vi "数据表比对.vi"(8 "error in (no error)":errorcluster, 9 "查询元素输入":string(combo), 10 "仪器日志参数":string, 11 "table输入":string(combo)) -> (0 "error out":errorcluster, 2 "待发送第一条数据":string[](array[string]), 3 "待发送数据":string[][](table))   [LabVIEW 2016, in "数据传输系统.lvlib"]
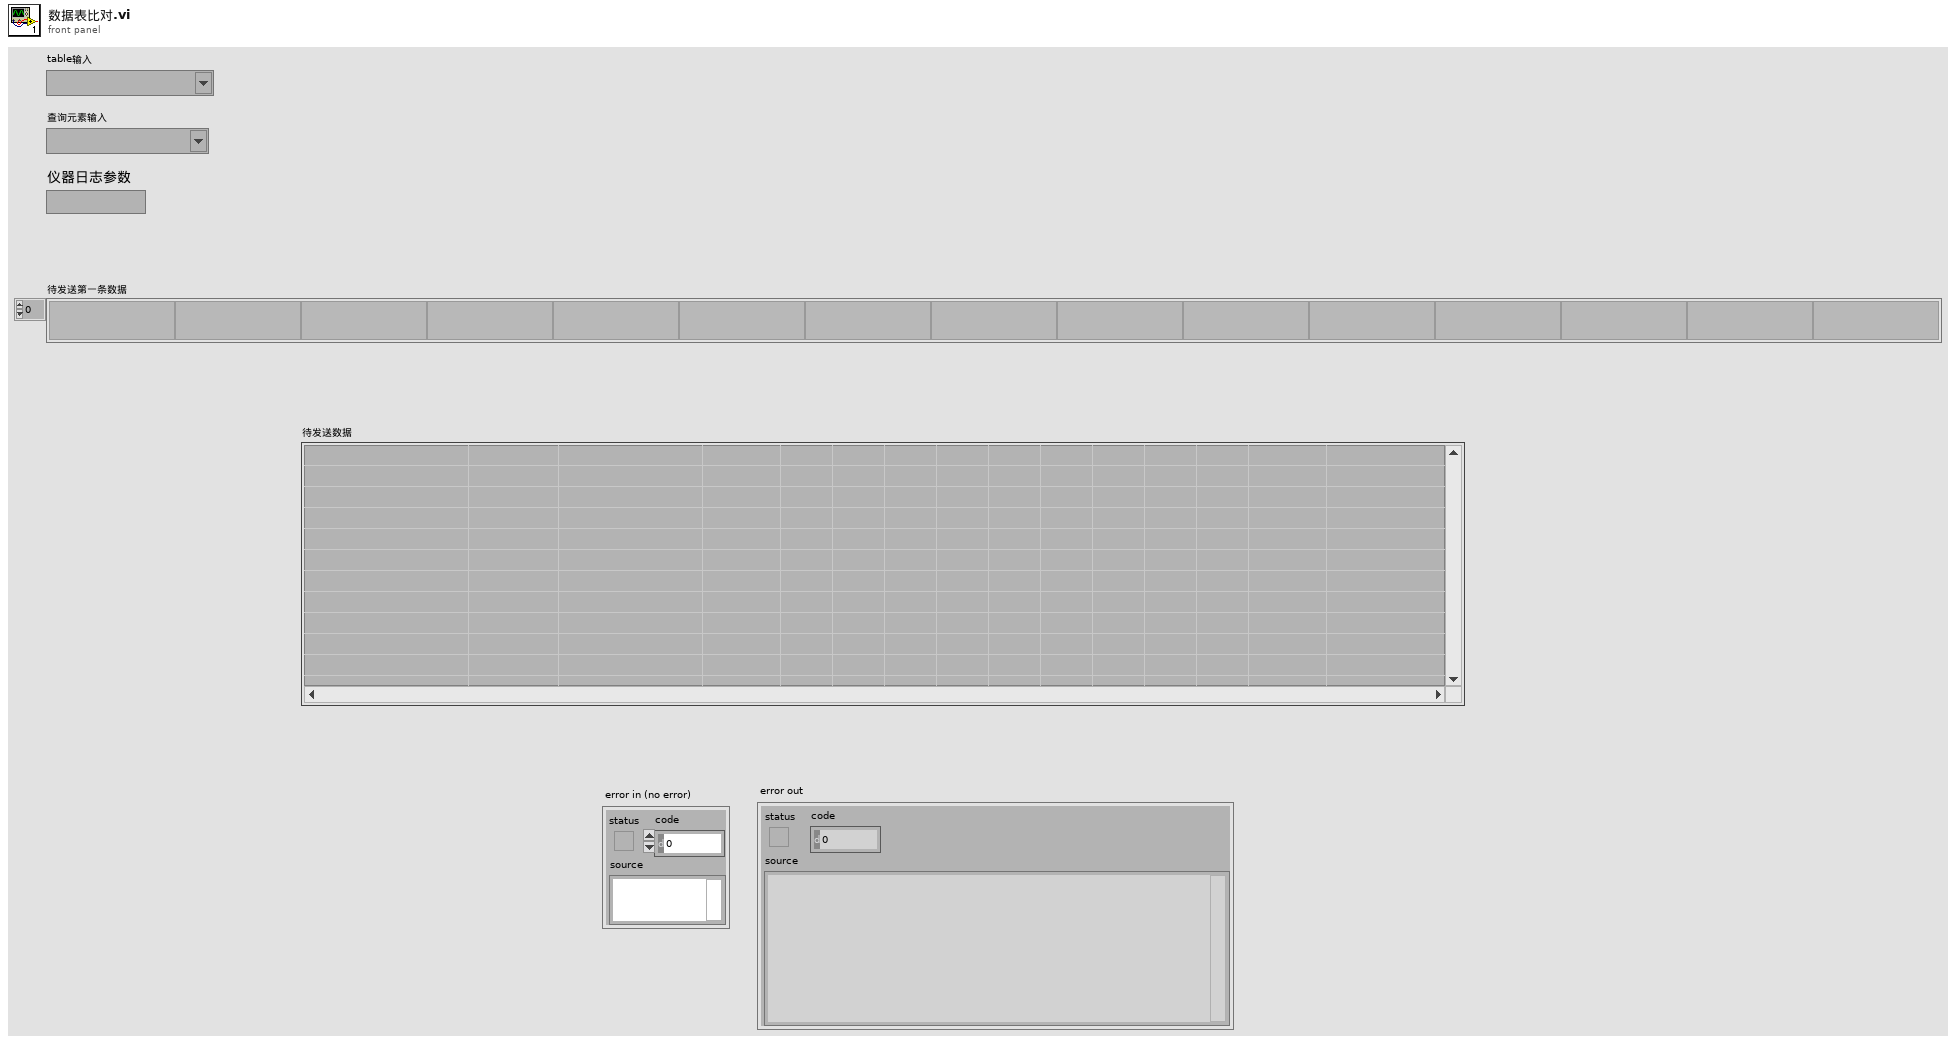
[diagram p1: front panel]
types:
  T1 = typedef "LVDateTimeRec.ctl" = cluster{"秒数的小数部分":dbl, "秒":i32, "分":i32, "时":i32, "日":i32, "月":i32, "年":i32, "天数（周）":i32, "天数（年）":i32, "DST":i32}
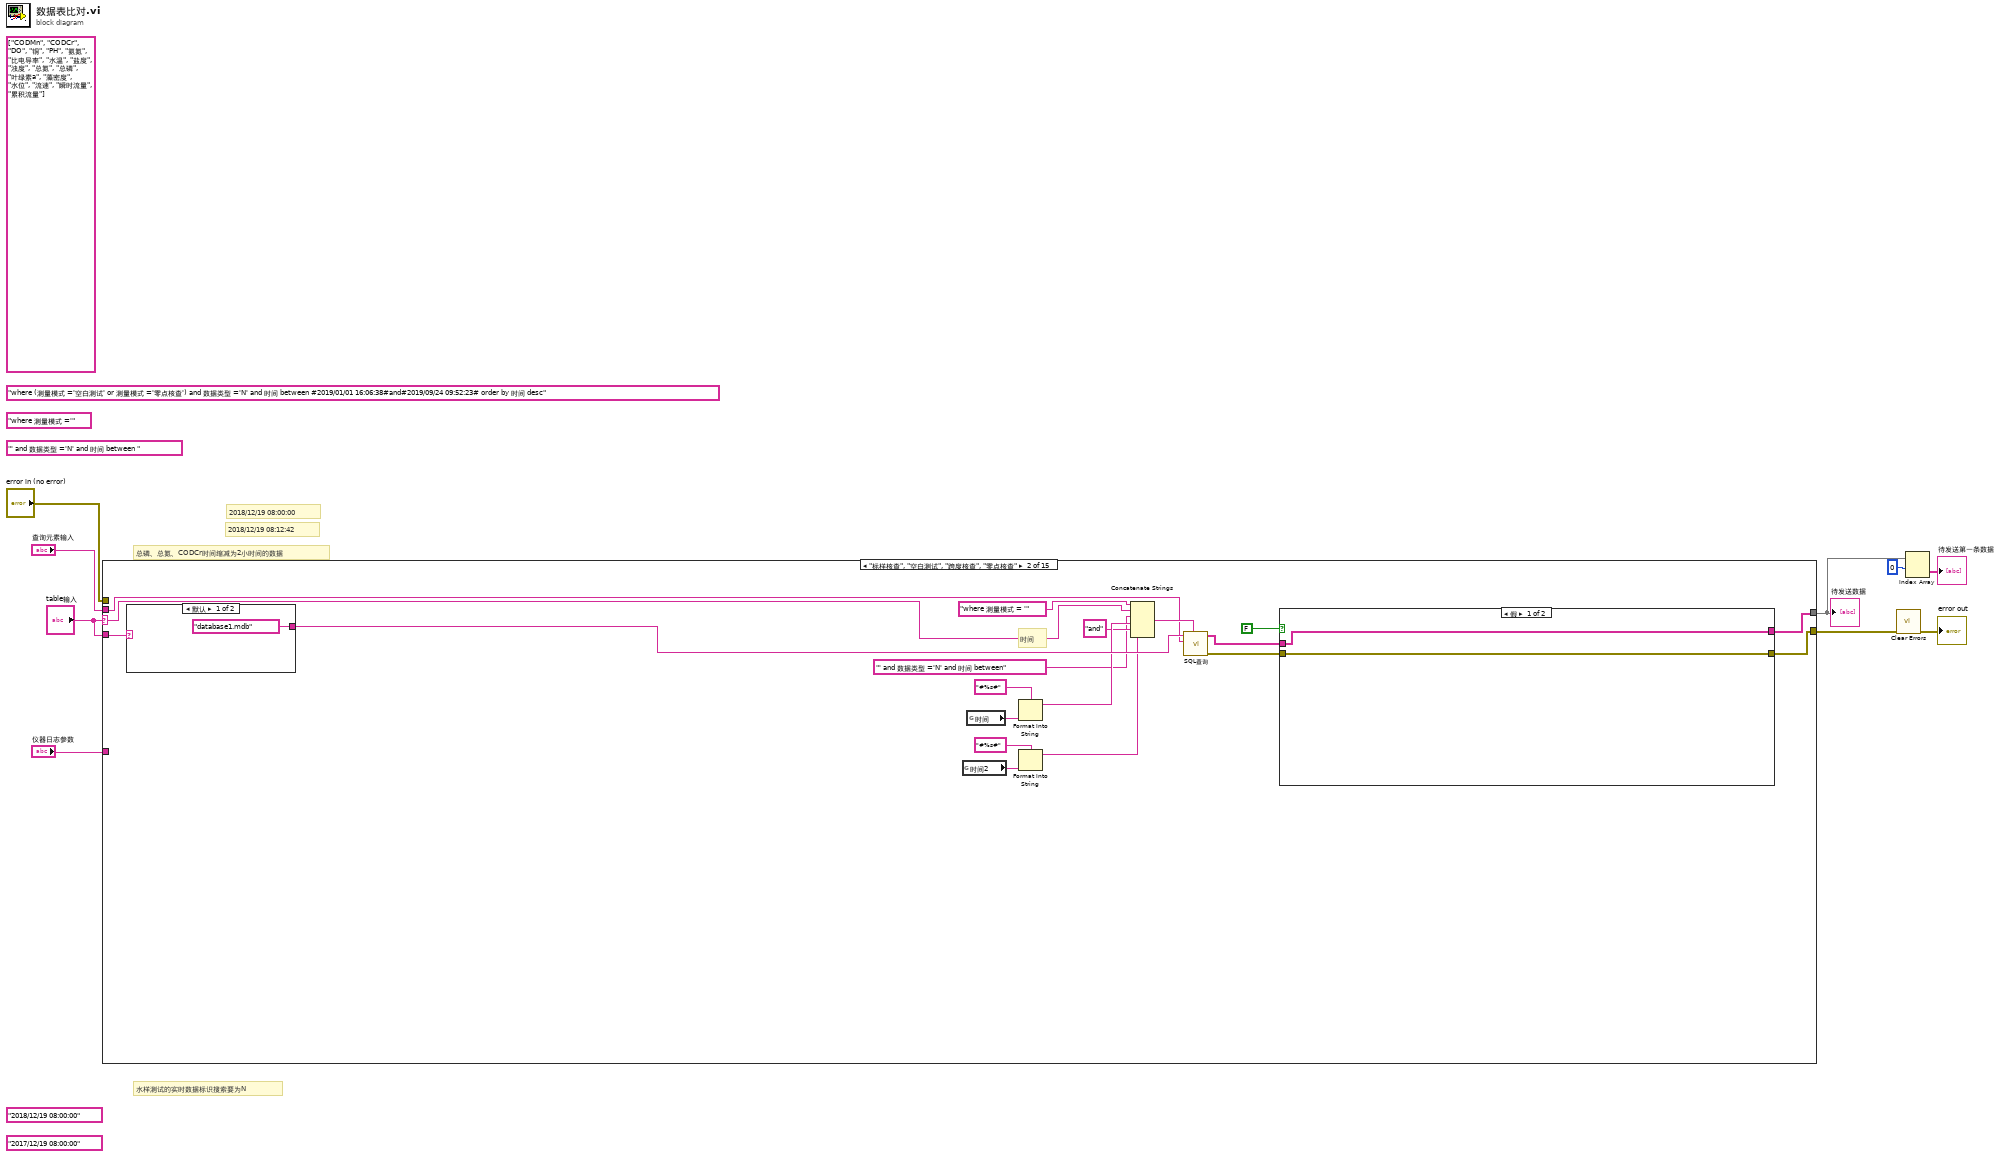
[diagram p0: block diagram]
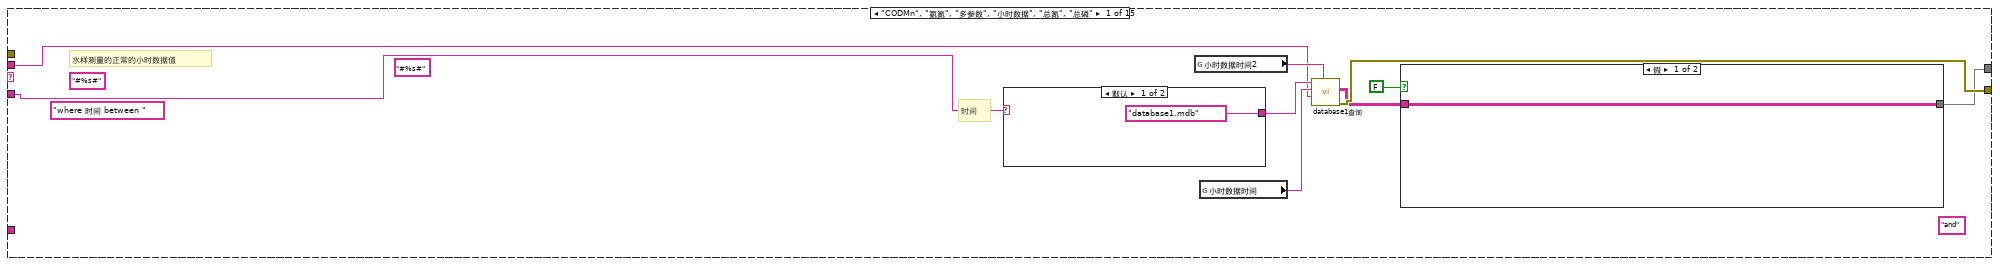
[diagram p2: hidden frame]
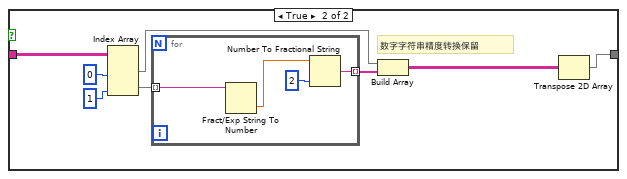
[diagram p3: hidden frame]
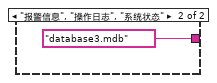
[diagram p4: hidden frame]
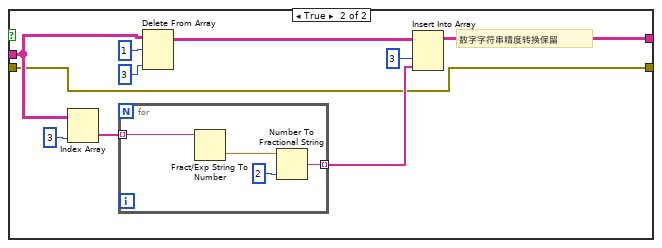
[diagram p5: hidden frame]
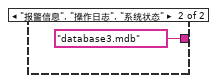
[diagram p6: hidden frame]
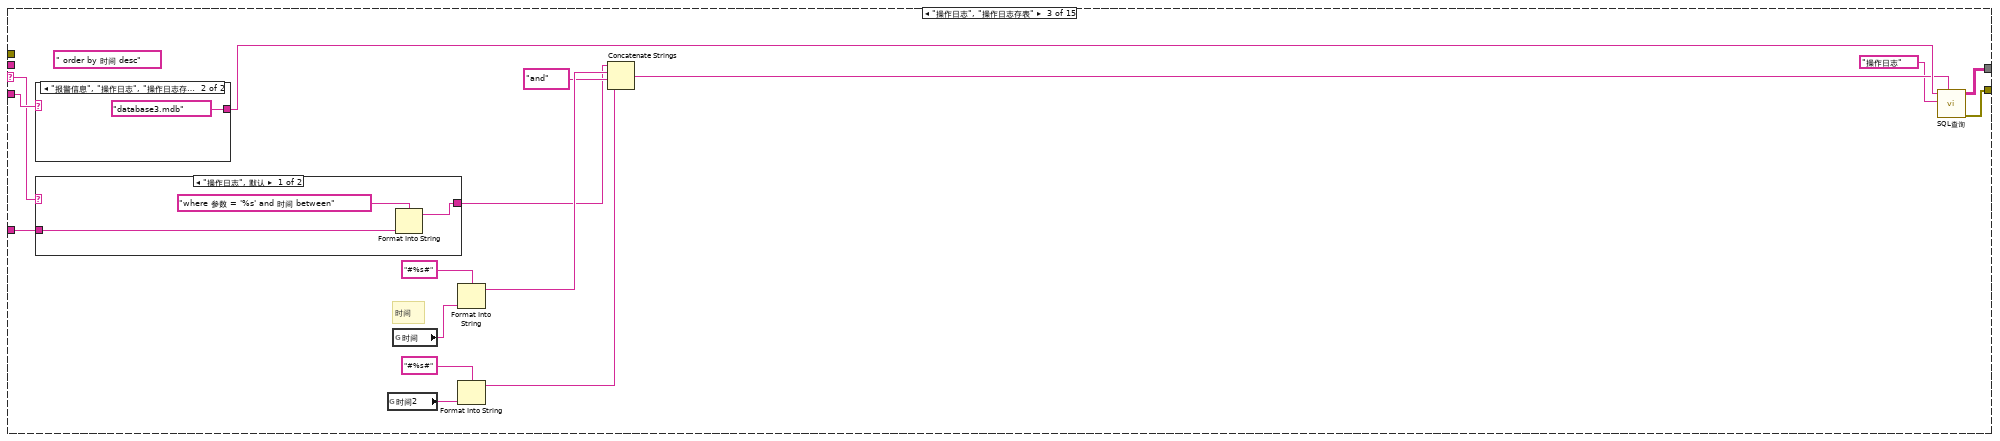
[diagram p7: hidden frame]
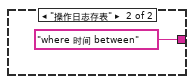
[diagram p8: hidden frame]
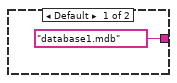
[diagram p9: hidden frame]
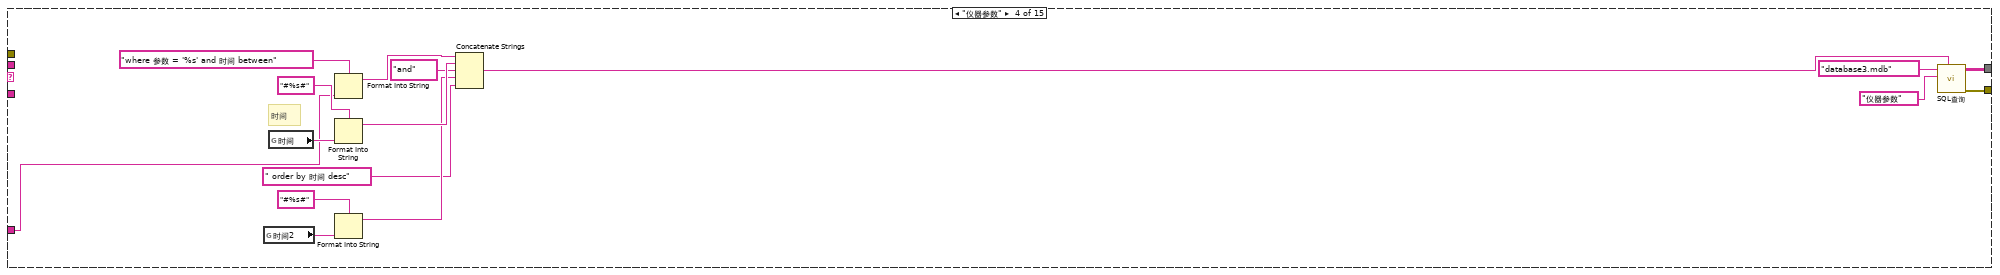
[diagram p10: hidden frame]
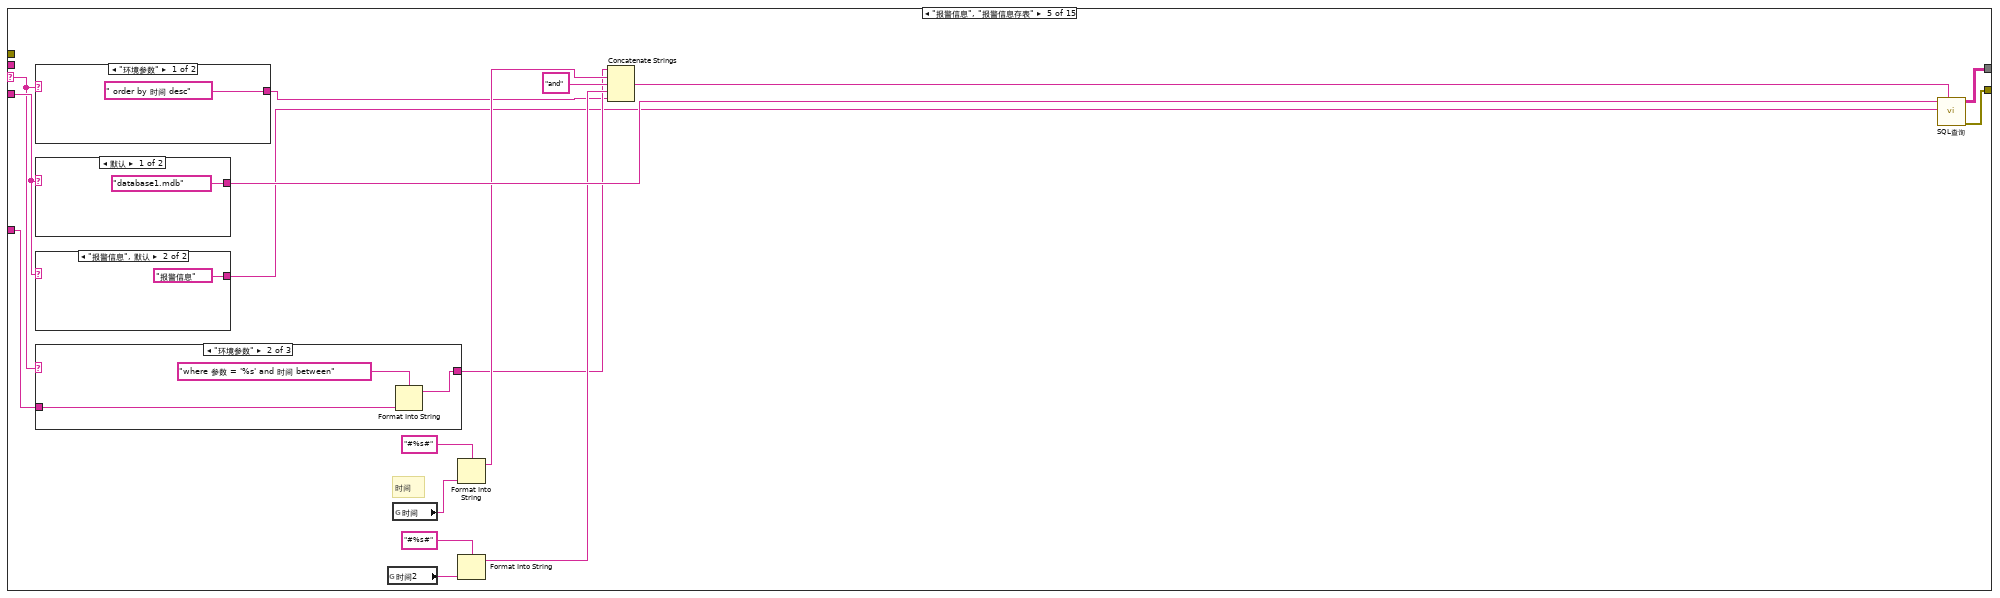
[diagram p11: hidden frame]
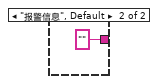
[diagram p12: hidden frame]
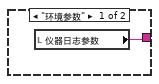
[diagram p13: hidden frame]
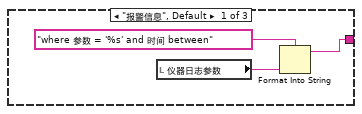
[diagram p14: hidden frame]
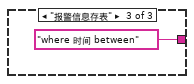
[diagram p15: hidden frame]
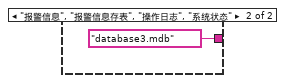
[diagram p16: hidden frame]
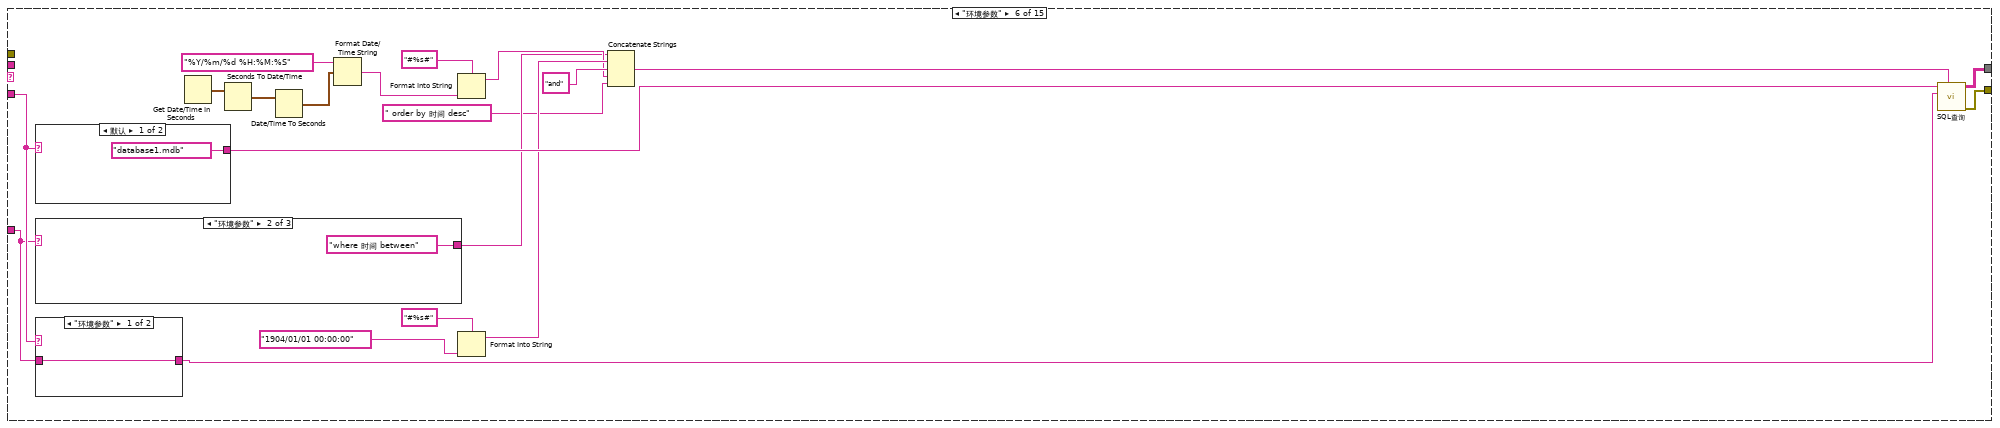
[diagram p17: hidden frame]
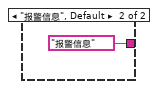
[diagram p18: hidden frame]
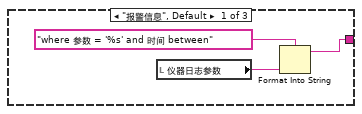
[diagram p19: hidden frame]
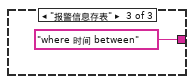
[diagram p20: hidden frame]
diagram:
  (unwired) "' and 数据类型 ='N' and 时间 between "
  (unwired) "where 测量模式 ='" ("condition")
  (unwired) "where (测量模式 ='空白测试' or 测量模式 ='零点核查') and 数据类型 ='N' and 时间 between #2019/01/01 16:06:38#and#2019/09/24 09:52:23# order by 时间 desc" ("condition")
  (unwired) string[] ["CODMn", "CODCr", "DO", "铜", "PH", "氨氮", "比电导率", "水温", "盐度", "浊度", "总氮", "总磷", "叶绿素a", "藻密度", "水位", "流速", "瞬时流量", "累积流量"] ("查询参数数组")
  (unwired) "2017/12/19 08:00:00"
  (unwired) "2018/12/19 08:00:00"
  # "水样测试的实时数据标识搜索要为N"
  # "2018/12/19 08:00:00"
  # "总磷、总氮、CODCr时间缩减为2小时间的数据"
  # "2018/12/19 08:12:42"
  n1 = case shown="\"标样核查\", \"空白测试\", \"跨度核查\", \"零点核查\"" "table输入" {
    selector: "table输入" -> [_ w35 w72 _ w109 _ _ _ _ _ _ _ _ _ _]
    tunnel: "error in (no error)" -> [_ _ _ _ _ _ w170 _ _ _ _ _ _ _ _]
    tunnel: [w16 w38 w84 w107 w124 w157 w170 w185 w281 w328 w382 w437 w480 w523 w564] -> w7
    tunnel: [w12 w41 w82 w105 w122 w155 w168 w188 w284 w331 w385 w440 w483 w526 w566] -> w3
    tunnel: "table输入" -> [w18 w52 w86 _ w112 w147 _ _ _ _ _ _ _ _ _]
    tunnel: "查询元素输入" -> [w10 w34 _ _ _ _ _ w171 w270 w317 w371 w430 w473 w516 w559]
    tunnel: "仪器日志参数" -> [_ _ w71 w93 w110 w139 _ _ _ _ _ _ _ _ _]
    frame "CODMn", "氨氮", "多参数", "小时数据", "总氮", "总磷" {
      (unwired) "and" ("字符串")
      (unwired) "#%s#" ("初始字符串")
      (unwired) "#%s#" ("初始字符串")
      (unwired) "where 时间 between " ("condition")
      # "水样测量的正常的小时数据值"
      # "时间"
      n2 = case shown="默认" w18 {
        tunnel: ["database1.mdb" ("database") "database3.mdb" ("database")] -> w17
        frame Default {
        }
        frame "报警信息", "操作日志", "系统状态" {
        }
      }
      n3 = global read "全局 时间2.vi" "小时数据时间2"() -> (w14:string)
      n4 = global read "全局 水样时间.vi" "小时数据时间"() -> (w15:string)
      n5 = call "database1查询.vi"("时间2"=w14, "table"=w10, "时间1"=w15, "database"=w17) -> ("error out"=w16:errorcluster, "data"=w13:string[][])  [unwired: 4 in, 1 out]
      n6 = case shown="假" FALSE {
        tunnel: w13 -> [w19 w27]
        tunnel: [w19 w20] -> w12
        frame False {
        }
        frame True {
          # "数字字符串精度转换保留"
          n7 = Index Array(array=w27, index (col) #1=0 ("禁用的索引 (列)"), index (col) #2=1 ("索引 (列)")) -> (element #1=w23:string[], element #2=w24:string[])  [unwired: 2 in]
          n8 = for {
            tunnel: w24 -> [w29] mode=indexing
            tunnel: [w28] -> w22 mode=indexing
            n9 = Fract/Exp String To Number(string=w29) -> (number=w30:dbl)  [unwired: 3 in, 1 out]
            n10 = Number To Fractional String(number=w30, precision (6)=i16 2 ("精度(6)")) -> (F-format string=w28:string)  [unwired: 2 in]
          }
          n11 = Build Array(w23, w22) -> (w21:string[][])
          n12 = Transpose 2D Array(2D array=w21) -> (transposed array=w20:string[][])
        }
      }
    }
    frame "标样核查", "空白测试", "跨度核查", "零点核查" {
      # "时间"
      n13 = case shown="默认" w52 {
        tunnel: ["database1.mdb" ("database") "database3.mdb" ("database")] -> w51
        frame Default {
        }
        frame "报警信息", "操作日志", "系统状态" {
        }
      }
      n14 = global read "全局 时间2.vi" "时间2"() -> (w43:string)
      n15 = global read "全局 水样时间.vi" "时间"() -> (w44:string)
      n16 = Format Into String(format string="#%s#" ("初始字符串"), w44) -> (resulting string=w50:string)  [unwired: 2 in, 1 out]
      n17 = Format Into String(format string="#%s#" ("初始字符串"), w43) -> (resulting string=w46:string)  [unwired: 2 in, 1 out]
      n18 = Concatenate Strings("where 测量模式 = '" ("condition"), w35, "' and 数据类型 ='N' and 时间 between" ("字符串"), w50, "and" ("字符串"), w46) -> (w45:string)
      n19 = call "SQL查询.vi"("condition"=w45, "table输入"=w34, "database"=w51) -> ("error out"=w39:errorcluster, "data"=w42:string[][])  [unwired: 7 in]
      n20 = case shown="假" FALSE {
        tunnel: w42 -> [w54 w57]
        tunnel: [w54 w56] -> w41
        tunnel: [w53 w55] -> w38
        tunnel: w39 -> [w53 w55]
        frame False {
        }
        frame True {
          # "数字字符串精度转换保留"
          n21 = Index Array(array=w57, index (col)=3 ("禁用的索引 (列)")) -> (element=w63:string[])  [unwired: 1 in]
          n22 = for {
            tunnel: w63 -> [w66] mode=indexing
            tunnel: [w65] -> w59 mode=indexing
            n23 = Fract/Exp String To Number(string=w66) -> (number=w67:dbl)  [unwired: 3 in, 1 out]
            n24 = Number To Fractional String(number=w67, precision (6)=i16 2 ("精度(6)")) -> (F-format string=w65:string)  [unwired: 2 in]
          }
          n25 = Delete From Array(array=w57, length=1 ("长度"), index (col)=3 ("禁用的索引 (列)")) -> (array with subset deleted=w60:string[][])  [unwired: 1 in, 1 out]
          n26 = Insert Into Array(array=w60, index (col)=3 ("禁用的索引 (列)"), new element=w59) -> (w56:string[][])  [unwired: 1 in]
        }
      }
    }
    frame "操作日志", "操作日志存表" {
      (unwired) " order by 时间 desc" ("字符串")
      # "时间"
      n27 = case shown="\"报警信息\", \"操作日志\", \"操作日志存表\", \"系统状态\"" w86 {
        tunnel: ["database1.mdb" ("database") "database3.mdb" ("database")] -> w85
        frame Default {
        }
        frame "报警信息", "操作日志", "操作日志存表", "系统状态" {
        }
      }
      n28 = case shown="\"操作日志\", 默认" w72 {
        tunnel: [w88 "where 时间 between" ("condition")] -> w74
        tunnel: w71 -> [w87 _]
        frame "操作日志", Default {
          n29 = Format Into String(format string="where 参数 = '%s' and 时间 between" ("condition"), w87) -> (resulting string=w88:string)  [unwired: 2 in, 1 out]
        }
        frame "操作日志存表" {
        }
      }
      n30 = global read "全局 时间2.vi" "时间2"() -> (w75:string)
      n31 = global read "全局 水样时间.vi" "时间"() -> (w76:string)
      n32 = Format Into String(format string="#%s#" ("初始字符串"), w76) -> (resulting string=w81:string)  [unwired: 2 in, 1 out]
      n33 = Format Into String(format string="#%s#" ("初始字符串"), w75) -> (resulting string=w77:string)  [unwired: 2 in, 1 out]
      n34 = Concatenate Strings(w74, w81, "and" ("字符串"), w77) -> (w83:string)
      n35 = call "SQL查询.vi"("condition"=w83, "table输入"="操作日志", "database"=w85) -> ("error out"=w84:errorcluster, "data"=w82:string[][])  [unwired: 7 in]
    }
    frame "仪器参数" {
      # "时间"
      n36 = global read "全局 时间2.vi" "时间2"() -> (w98:string)
      n37 = global read "全局 水样时间.vi" "时间"() -> (w99:string)
      n38 = Format Into String(format string="where 参数 = '%s' and 时间 between" ("condition"), w93) -> (resulting string=w97:string)  [unwired: 2 in, 1 out]
      n39 = Format Into String(format string="#%s#" ("初始字符串"), w99) -> (resulting string=w104:string)  [unwired: 2 in, 1 out]
      n40 = Format Into String(format string="#%s#" ("初始字符串"), w98) -> (resulting string=w100:string)  [unwired: 2 in, 1 out]
      n41 = Concatenate Strings(w97, w104, "and" ("字符串"), w100, " order by 时间 desc" ("字符串")) -> (w106:string)
      n42 = call "SQL查询.vi"("condition"=w106, "table输入"="仪器参数", "database"="database3.mdb") -> ("error out"=w107:errorcluster, "data"=w105:string[][])  [unwired: 7 in]
    }
    frame "报警信息", "报警信息存表" {
      # "时间"
      n43 = case shown="\"环境参数\"" w109 {
        tunnel: [" order by 时间 desc" ("字符串") "" ("仪器日志参数")] -> w111
        frame "环境参数" {
        }
        frame "报警信息", Default {
        }
      }
      n44 = case shown="默认" w112 {
        tunnel: ["database1.mdb" ("database") "database3.mdb" ("database")] -> w125
        frame Default {
        }
        frame "报警信息", "报警信息存表", "操作日志", "系统状态" {
        }
      }
      n45 = case shown="\"报警信息\", 默认" w112 {
        tunnel: [w128 "报警信息" ("table输入")] -> w113
        frame "环境参数" {
          n46 = local read "仪器日志参数"() -> (w128:string)
        }
        frame "报警信息", Default {
        }
      }
      n47 = case shown="\"环境参数\"" w109 {
        tunnel: [w131 w134 "where 时间 between" ("condition")] -> w114
        tunnel: w110 -> [_ w133 _]
        frame "报警信息", Default {
          n48 = local read "仪器日志参数"() -> (w130:string)
          n49 = Format Into String(format string="where 参数 = '%s' and 时间 between" ("condition"), w130) -> (resulting string=w131:string)  [unwired: 2 in, 1 out]
        }
        frame "环境参数" {
          n50 = Format Into String(format string="where 参数 = '%s' and 时间 between" ("condition"), w133) -> (resulting string=w134:string)  [unwired: 2 in, 1 out]
        }
        frame "报警信息存表" {
        }
      }
      n51 = global read "全局 时间2.vi" "时间2"() -> (w115:string)
      n52 = global read "全局 水样时间.vi" "时间"() -> (w116:string)
      n53 = Format Into String(format string="#%s#" ("初始字符串"), w116) -> (resulting string=w121:string)  [unwired: 2 in, 1 out]
      n54 = Format Into String(format string="#%s#" ("初始字符串"), w115) -> (resulting string=w117:string)  [unwired: 2 in, 1 out]
      n55 = Concatenate Strings(w114, w121, "and" ("字符串"), w117, w111) -> (w123:string)
      n56 = call "SQL查询.vi"("condition"=w123, "table输入"=w113, "database"=w125) -> ("error out"=w124:errorcluster, "data"=w122:string[][])  [unwired: 7 in]
    }
    frame "环境参数" {
      n57 = case shown="默认" w147 {
        tunnel: ["database1.mdb" ("database") "database3.mdb" ("database")] -> w158
        frame Default {
        }
        frame "报警信息", "报警信息存表", "操作日志", "系统状态" {
        }
      }
      n58 = case shown="\"环境参数\"" w139 {
        tunnel: [w162 "where 时间 between" ("condition") "where 时间 between" ("condition")] -> w149
        frame "报警信息", Default {
          n59 = local read "仪器日志参数"() -> (w161:string)
          n60 = Format Into String(format string="where 参数 = '%s' and 时间 between" ("condition"), w161) -> (resulting string=w162:string)  [unwired: 2 in, 1 out]
        }
        frame "环境参数" {
        }
        frame "报警信息存表" {
        }
      }
      n61 = case shown="\"环境参数\"" w147 {
        tunnel: [w159 "报警信息" ("table输入")] -> w148
        tunnel: w139 -> [w159 _]
        frame "环境参数" {
        }
        frame "报警信息", Default {
        }
      }
      n62 = Get Date/Time In Seconds() -> (seconds since 1Jan1904=w144:timestamp)
      n63 = Seconds To Date/Time(time stamp (now)=w144) -> (date time rec=w141:T1)  [unwired: 1 in]
      n64 = Date/Time To Seconds(2:w141) -> (0:w143:timestamp)  [unwired: 1 in]
      n65 = Format Date/Time String(time format string (%c)="%Y/%m/%d %H:%M:%S" ("时间格式字符串(%c)"), seconds (now)=w143) -> (date/time string=w140:string)  [unwired: 1 in]
      n66 = Format Into String(format string="#%s#" ("初始字符串"), w140) -> (resulting string=w150:string)  [unwired: 2 in, 1 out]
      n67 = Format Into String(format string="#%s#" ("初始字符串"), "1904/01/01 00:00:00") -> (resulting string=w154:string)  [unwired: 2 in, 1 out]
      n68 = Concatenate Strings(w149, w154, "and" ("字符串"), w150, " order by 时间 desc" ("字符串")) -> (w156:string)
      n69 = call "SQL查询.vi"("condition"=w156, "table输入"=w148, "database"=w158) -> ("error out"=w157:errorcluster, "data"=w155:string[][])  [unwired: 7 in]
    }
    frame Default {
      # "时间格式转换"
      n70 = local read "待发送数据"() -> (w169:string[][])
      n71 = call "数组时间戳格式化(子VI).vi"("待发送数据输入"=w169) -> ("待发送数据输出"=w168:string[][])  [unwired: 10 in]
    }
    frame "实时数据" {
      (unwired) " order by 时间 desc" ("字符串")
      # "空白测试or零点核查要加括号"
      # "上传本地时间点的实时数据"
      # "上传质控数据（空白测试，跨度核查，核查数据，平行样数据）"
      n72 = global read "全局 实时数据参数.vi" "实时数据参数"() -> (w181:string)
      n73 = case shown="\"空白测试\"" w181 {
        tunnel: [w205 w227 w238 w244] -> w182
        tunnel: w181 -> [w201 w226 _ w240]
        tunnel: [w204 w222 w234 w239] -> w176
        tunnel: w171 -> [_ w221 _ _]
        frame "水样测试" {
          n74 = Get Date/Time In Seconds() -> (seconds since 1Jan1904=w213:timestamp)
          n75 = Format Date/Time String(time format string (%c)="%Y%m%d%H%M%S%3u" ("时间格式字符串(%c)"), seconds (now)=w213) -> (date/time string=w211:string)  [unwired: 1 in]
          n76 = local read "查询元素输入"() -> (w206:string)
          n77 = Concatenate Strings("where 测量模式 ='" ("condition"), w201, "' and 数据类型 ='N' and 时间 between ") -> (w204:string)
          n78 = Replace Substring(2:8 ("长度（子字符串长度）"), 3:10 ("偏移量(0)"), 4:"0000" ("子字符串(\"\")"), 5:w211) -> (1:w207:string)  [unwired: 1 out]
          n79 = case shown="默认" w206 {
            tunnel: w207 -> [w215 w218 _]
            tunnel: [w214 w219 w220] -> w205
            frame Default {
              n80 = Search and Replace String(input string=w215, search string="." ("搜索字符串")) -> (result string=w216:string)  [unwired: 6 in, 3 out]
              n81 = call "格式时间字符串.vi"("字符串"=w216) -> ("连接的字符串"=w214:string)  [unwired: 10 in]
            }
            frame "CODCr", "CODMn", "累积流量", "总氮", "总磷" {
              n82 = call "实时数据查询用2小时间的数据.vi"("字符串"=w218) -> ("连接的字符串"=w219:string)  [unwired: 10 in]
            }
            frame "CODCr加标回收率", "CODMn加标回收率", "氨氮加标回收率", "总氮加标回收率", "总磷加标回收率" {
              n83 = global read "全局 时间2.vi" "加标回收索引起始时间"() -> (w220:string)
            }
          }
        }
        frame "空白测试" {
          n84 = case shown="\"氨氮\"" w221 {
            tunnel: [w228 w229 w230 w231 w232 w233] -> w227
            frame "CODMn" {
              n85 = global read "全局 时间2.vi" "CODMn零点核查索引起始时间"() -> (w228:string)
            }
            frame "CODCr" {
              n86 = global read "全局 时间2.vi" "CODCr零点核查索引起始时间"() -> (w229:string)
            }
            frame "氨氮" {
              n87 = global read "全局 时间2.vi" "氨氮零点核查索引起始时间"() -> (w230:string)
            }
            frame "总磷" {
              n88 = global read "全局 时间2.vi" "总磷零点核查索引起始时间"() -> (w231:string)
            }
            frame "总氮" {
              n89 = global read "全局 时间2.vi" "总氮零点核查索引起始时间"() -> (w232:string)
            }
            frame "", Default {
              n90 = global read "全局 时间2.vi" "零点核查索引起始时间"() -> (w233:string)
            }
          }
          n91 = Concatenate Strings("where (测量模式 ='" ("condition"), w226, "' or 测量模式 = '零点核查", "') and 数据类型 ='N' and 时间 between ") -> (w222:string)
        }
        frame "核查数据" {
          n92 = global read "全局 时间2.vi" "标样核查索引起始时间"() -> (w238:string)
          n93 = Concatenate Strings("where 测量模式 ='" ("condition"), "标样核查" ("实时数据参数"), "' and 数据类型 ='N' and 时间 between ") -> (w234:string)
        }
        frame "跨度核查", Default {
          n94 = local read "查询元素输入"() -> (w243:string)
          n95 = Concatenate Strings("where 测量模式 ='" ("condition"), w240, "' and 数据类型 ='N' and 时间 between ") -> (w239:string)
          n96 = case shown="\"氨氮\"" w243 {
            tunnel: [w245 w246 w247 w248 w249 w250] -> w244
            frame "CODMn" {
              n97 = global read "全局 时间2.vi" "CODMn跨度核查索引起始时间"() -> (w245:string)
            }
            frame "CODCr" {
              n98 = global read "全局 时间2.vi" "CODCr跨度核查索引起始时间"() -> (w246:string)
            }
            frame "氨氮" {
              n99 = global read "全局 时间2.vi" "氨氮跨度核查索引起始时间"() -> (w247:string)
            }
            frame "总磷" {
              n100 = global read "全局 时间2.vi" "总磷跨度核查索引起始时间"() -> (w248:string)
            }
            frame "总氮" {
              n101 = global read "全局 时间2.vi" "总氮跨度核查索引起始时间"() -> (w249:string)
            }
            frame "", Default {
              n102 = global read "全局 时间2.vi" "跨度核查索引起始时间"() -> (w250:string)
            }
          }
        }
      }
      n103 = global read "断电保存全局.vi" "数据组合发送"() -> (w173:bool)
      n104 = Get Date/Time In Seconds() -> (seconds since 1Jan1904=w180:timestamp)
      n105 = Seconds To Date/Time(time stamp (now)=w180) -> (date time rec=w175:T1)  [unwired: 1 in]
      n106 = case shown="真" w173 {
        tunnel: w175 -> [w195 w198]
        tunnel: [w195 w196] -> w174
        frame False {
        }
        frame True {
          n107 = Unbundle By Name(w198) -> ("时"=w200:i32)
          n108 = Subtract(x=w200, y=2) -> (x-y=w197:i32)
          n109 = Bundle By Name(cluster=w198, "时"=w197) -> (w196:T1)
        }
      }
      n110 = Date/Time To Seconds(2:w174) -> (0:w179:timestamp)  [unwired: 1 in]
      n111 = Format Date/Time String(time format string (%c)="%Y/%m/%d %H:%M:%S" ("时间格式字符串(%c)"), seconds (now)=w179) -> (date/time string=w177:string)  [unwired: 1 in]
      n112 = Format Into String(format string="#%s#" ("初始字符串"), w182) -> (resulting string=w194:string)  [unwired: 2 in, 1 out]
      n113 = Format Into String(format string="#%s#" ("初始字符串"), w177) -> (resulting string=w190:string)  [unwired: 2 in, 1 out]
      n114 = Concatenate Strings(w176, w194, "and" ("字符串"), w190, " order by 时间 asc" ("字符串")) -> (w184:string)
      n115 = call "SQL查询.vi"("condition"=w184, "table输入"=w171, "database"="database1.mdb") -> ("error out"=w186:errorcluster, "data"=w183:string[][])  [unwired: 7 in]
      n116 = case shown="\"CODCr\", \"总氮\", \"总磷\"" w171 {
        tunnel: w171 -> [_ w253]
        tunnel: w184 -> [_ w252]
        tunnel: w183 -> [_ w251]
        frame Default {
        }
        frame "CODCr", "总氮", "总磷" {
          n117 = global write "全局 实时数据参数.vi" "data"(w251) -> ()
          n118 = global write "全局 实时数据参数.vi" "参数"(w253) -> ()
          n119 = global write "全局 实时数据参数.vi" "连接的字符串"(w252) -> ()
        }
      }
      n120 = case shown="假" FALSE {
        tunnel: [w255 w258] -> w188
        tunnel: w183 -> [w255 w257]
        tunnel: w186 -> [w254 w256]
        tunnel: [w254 w256] -> w185
        frame False {
        }
        frame True {
          # "数字字符串精度转换保留"
          n121 = Index Array(array=w257, index (col)=3 ("禁用的索引 (列)")) -> (element=w264:string[])  [unwired: 1 in]
          n122 = for {
            tunnel: w264 -> [w267] mode=indexing
            tunnel: [w266] -> w260 mode=indexing
            n123 = Fract/Exp String To Number(string=w267) -> (number=w268:dbl)  [unwired: 3 in, 1 out]
            n124 = Number To Fractional String(number=w268, precision (6)=i16 2 ("精度(6)")) -> (F-format string=w266:string)  [unwired: 2 in]
          }
          n125 = Delete From Array(array=w257, length=1 ("长度"), index (col)=3 ("禁用的索引 (列)")) -> (array with subset deleted=w261:string[][])  [unwired: 1 in, 1 out]
          n126 = Insert Into Array(array=w261, index (col)=3 ("禁用的索引 (列)"), new element=w260) -> (w258:string[][])  [unwired: 1 in]
        }
      }
    }
    frame "加标回收" {
      w276 = "加标回收率" ("字符串")
      # "上传本地时间点的实时数据"
      # "上传加标回收数据"
      n127 = global read "全局 数据发送重叠.vi" "掉线指示灯"() -> (w277:bool)
      n128 = case shown="假" w277 {
        tunnel: [w293 w297] -> w278
        frame False {
          n129 = global read "全局 数据发送重叠.vi" "数据发送重叠"() -> (w294:bool)
          n130 = case shown="假" w294 {
            tunnel: [w295 w296] -> w293
            frame False {
              n131 = global read "全局 时间2.vi" "加标回收索引起始时间"() -> (w295:string)
            }
            frame True {
              n132 = global read "全局 数据发送重叠.vi" "数据发送重叠开始时间戳"() -> (w296:string)
            }
          }
        }
        frame True {
          n133 = global read "全局 数据发送重叠.vi" "TCP掉线时间节点"() -> (w297:string)
        }
      }
      n134 = Get Date/Time In Seconds() -> (seconds since 1Jan1904=w275:timestamp)
      n135 = Seconds To Date/Time(time stamp (now)=w275) -> (date time rec=w272:T1)  [unwired: 1 in]
      n136 = Date/Time To Seconds(2:w272) -> (0:w274:timestamp)  [unwired: 1 in]
      n137 = Format Date/Time String(time format string (%c)="%Y/%m/%d %H:%M:%S" ("时间格式字符串(%c)"), seconds (now)=w274) -> (date/time string=w271:string)  [unwired: 1 in]
      n138 = Format Into String(format string="#%s#" ("初始字符串"), w278) -> (resulting string=w292:string)  [unwired: 2 in, 1 out]
      n139 = Format Into String(format string="#%s#" ("初始字符串"), w271) -> (resulting string=w288:string)  [unwired: 2 in, 1 out]
      n140 = Concatenate Strings("where 参数 ='" ("condition"), w270, "' and 时间 between ", w292, "and" ("字符串"), w288) -> (w280:string)
      n141 = call "SQL查询.vi"("condition"=w280, "table输入"=w276, "database"="database1.mdb") -> ("error out"=w282:errorcluster, "data"=w279:string[][])  [unwired: 7 in]
      n142 = case shown="\"CODCr\", \"总氮\", \"总磷\"" w276 {
        tunnel: w276 -> [_ w300]
        tunnel: w280 -> [_ w299]
        tunnel: w279 -> [_ w298]
        frame Default {
        }
        frame "CODCr", "总氮", "总磷" {
          n143 = global write "全局 实时数据参数.vi" "data"(w298) -> ()
          n144 = global write "全局 实时数据参数.vi" "参数"(w300) -> ()
          n145 = global write "全局 实时数据参数.vi" "连接的字符串"(w299) -> ()
        }
      }
      n146 = case shown="假" FALSE {
        tunnel: [w302 w305] -> w284
        tunnel: w279 -> [w302 w304]
        tunnel: w282 -> [w301 w303]
        tunnel: [w301 w303] -> w281
        frame False {
        }
        frame True {
          # "数字字符串精度转换保留"
          n147 = Index Array(array=w304, index (col)=3 ("禁用的索引 (列)")) -> (element=w311:string[])  [unwired: 1 in]
          n148 = for {
            tunnel: w311 -> [w314] mode=indexing
            tunnel: [w313] -> w307 mode=indexing
            n149 = Fract/Exp String To Number(string=w314) -> (number=w315:dbl)  [unwired: 3 in, 1 out]
            n150 = Number To Fractional String(number=w315, precision (6)=i16 2 ("精度(6)")) -> (F-format string=w313:string)  [unwired: 2 in]
          }
          n151 = Delete From Array(array=w304, length=1 ("长度"), index (col)=3 ("禁用的索引 (列)")) -> (array with subset deleted=w308:string[][])  [unwired: 1 in, 1 out]
          n152 = Insert Into Array(array=w308, index (col)=3 ("禁用的索引 (列)"), new element=w307) -> (w305:string[][])  [unwired: 1 in]
        }
      }
    }
    frame "平行样测试" {
      w323 = "平行样测试" ("字符串")
      # "上传本地时间点的实时数据"
      # "上传平行样数据"
      n153 = global read "全局 数据发送重叠.vi" "掉线指示灯"() -> (w324:bool)
      n154 = case shown="假" w324 {
        tunnel: [w340 w351] -> w325
        frame False {
          n155 = global read "全局 数据发送重叠.vi" "数据发送重叠"() -> (w341:bool)
          n156 = case shown="假" w341 {
            tunnel: [w342 w350] -> w340
            frame False {
              n157 = local read "查询元素输入"() -> (w343:string)
              n158 = case shown="\"CODCr\"" w343 {
                tunnel: [w344 w345 w346 w347 w348 w349] -> w342
                frame "CODMn" {
                  n159 = global read "全局 时间2.vi" "CODMn平行样索引起始时间"() -> (w344:string)
                }
                frame "CODCr" {
                  n160 = global read "全局 时间2.vi" "CODCr平行样索引起始时间"() -> (w345:string)
                }
                frame "氨氮" {
                  n161 = global read "全局 时间2.vi" "氨氮平行样索引起始时间"() -> (w346:string)
                }
                frame "总磷" {
                  n162 = global read "全局 时间2.vi" "总磷平行样索引起始时间"() -> (w347:string)
                }
                frame "总氮" {
                  n163 = global read "全局 时间2.vi" "总磷平行样索引起始时间"() -> (w348:string)
                }
                frame "", Default {
                  n164 = global read "全局 时间2.vi" "平行样索引起始时间"() -> (w349:string)
                }
              }
            }
            frame True {
              n165 = global read "全局 数据发送重叠.vi" "数据发送重叠开始时间戳"() -> (w350:string)
            }
          }
        }
        frame True {
          n166 = global read "全局 数据发送重叠.vi" "TCP掉线时间节点"() -> (w351:string)
        }
      }
      n167 = Get Date/Time In Seconds() -> (seconds since 1Jan1904=w322:timestamp)
      n168 = Seconds To Date/Time(time stamp (now)=w322) -> (date time rec=w319:T1)  [unwired: 1 in]
      n169 = Date/Time To Seconds(2:w319) -> (0:w321:timestamp)  [unwired: 1 in]
      n170 = Format Date/Time String(time format string (%c)="%Y/%m/%d %H:%M:%S" ("时间格式字符串(%c)"), seconds (now)=w321) -> (date/time string=w318:string)  [unwired: 1 in]
      n171 = Format Into String(format string="#%s#" ("初始字符串"), w325) -> (resulting string=w339:string)  [unwired: 2 in, 1 out]
      n172 = Format Into String(format string="#%s#" ("初始字符串"), w318) -> (resulting string=w335:string)  [unwired: 2 in, 1 out]
      n173 = Concatenate Strings("where 参数 ='" ("condition"), w317, "' and 时间 between ", w339, "and" ("字符串"), w335) -> (w327:string)
      n174 = call "SQL查询.vi"("condition"=w327, "table输入"=w323, "database"="database1.mdb") -> ("error out"=w329:errorcluster, "data"=w326:string[][])  [unwired: 7 in]
      n175 = case shown="默认" w323 {
        tunnel: w323 -> [_ w354]
        tunnel: w327 -> [_ w353]
        tunnel: w326 -> [_ w352]
        frame Default {
        }
        frame "CODCr", "总氮", "总磷" {
          n176 = global write "全局 实时数据参数.vi" "data"(w352) -> ()
          n177 = global write "全局 实时数据参数.vi" "参数"(w354) -> ()
          n178 = global write "全局 实时数据参数.vi" "连接的字符串"(w353) -> ()
        }
      }
      n179 = case shown="假" FALSE {
        tunnel: [w356 w359] -> w331
        tunnel: w326 -> [w356 w358]
        tunnel: w329 -> [w355 w357]
        tunnel: [w355 w357] -> w328
        frame False {
        }
        frame True {
          # "数字字符串精度转换保留"
          n180 = Index Array(array=w358, index (col)=3 ("禁用的索引 (列)")) -> (element=w365:string[])  [unwired: 1 in]
          n181 = for {
            tunnel: w365 -> [w368] mode=indexing
            tunnel: [w367] -> w361 mode=indexing
            n182 = Fract/Exp String To Number(string=w368) -> (number=w369:dbl)  [unwired: 3 in, 1 out]
            n183 = Number To Fractional String(number=w369, precision (6)=i16 2 ("精度(6)")) -> (F-format string=w367:string)  [unwired: 2 in]
          }
          n184 = Delete From Array(array=w358, length=1 ("长度"), index (col)=3 ("禁用的索引 (列)")) -> (array with subset deleted=w362:string[][])  [unwired: 1 in, 1 out]
          n185 = Insert Into Array(array=w362, index (col)=3 ("禁用的索引 (列)"), new element=w361) -> (w359:string[][])  [unwired: 1 in]
        }
      }
    }
    frame "集成干预测试" {
      w377 = "集成干预测试" ("字符串")
      # "上传本地时间点的实时数据"
      # "上传集成干预数据"
      n186 = global read "全局 数据发送重叠.vi" "掉线指示灯"() -> (w378:bool)
      n187 = case shown="假" w378 {
        tunnel: [w394 w410] -> w379
        frame False {
          n188 = global read "全局 数据发送重叠.vi" "数据发送重叠"() -> (w395:bool)
          n189 = case shown="假" w395 {
            tunnel: [w396 w409] -> w394
            frame False {
              n190 = local read "查询元素输入"() -> (w397:string)
              n191 = case shown="\"浊度\"" w397 {
                tunnel: [w398 w399 w400 w401 w402 w403 w404 w405 w406 w407 w408] -> w396
                frame "CODMn" {
                  n192 = global read "全局 时间2.vi" "CODMn集成干预索引起始时间"() -> (w398:string)
                }
                frame "CODCr" {
                  n193 = global read "全局 时间2.vi" "CODCr集成干预索引起始时间"() -> (w399:string)
                }
                frame "氨氮" {
                  n194 = global read "全局 时间2.vi" "氨氮集成干预索引起始时间"() -> (w400:string)
                }
                frame "总磷" {
                  n195 = global read "全局 时间2.vi" "总磷集成干预索引起始时间"() -> (w401:string)
                }
                frame "总氮" {
                  n196 = global read "全局 时间2.vi" "总氮集成干预索引起始时间"() -> (w402:string)
                }
                frame "DO" {
                  n197 = global read "全局 时间2.vi" "DO集成干预索引起始时间"() -> (w403:string)
                }
                frame "PH" {
                  n198 = global read "全局 时间2.vi" "PH集成干预索引起始时间"() -> (w404:string)
                }
                frame "比电导率" {
                  n199 = global read "全局 时间2.vi" "比电导率集成干预索引起始时间"() -> (w405:string)
                }
                frame "水温" {
                  n200 = global read "全局 时间2.vi" "水温集成干预索引起始时间"() -> (w406:string)
                }
                frame "浊度" {
                  n201 = global read "全局 时间2.vi" "浊度集成干预索引起始时间"() -> (w407:string)
                }
                frame "", Default {
                  n202 = global read "全局 时间2.vi" "平行样索引起始时间"() -> (w408:string)
                }
              }
            }
            frame True {
              n203 = global read "全局 数据发送重叠.vi" "数据发送重叠开始时间戳"() -> (w409:string)
            }
          }
        }
        frame True {
          n204 = global read "全局 数据发送重叠.vi" "TCP掉线时间节点"() -> (w410:string)
        }
      }
      n205 = Get Date/Time In Seconds() -> (seconds since 1Jan1904=w376:timestamp)
      n206 = Seconds To Date/Time(time stamp (now)=w376) -> (date time rec=w373:T1)  [unwired: 1 in]
      n207 = Date/Time To Seconds(2:w373) -> (0:w375:timestamp)  [unwired: 1 in]
      n208 = Format Date/Time String(time format string (%c)="%Y/%m/%d %H:%M:%S" ("时间格式字符串(%c)"), seconds (now)=w375) -> (date/time string=w372:string)  [unwired: 1 in]
      n209 = Format Into String(format string="#%s#" ("初始字符串"), w379) -> (resulting string=w393:string)  [unwired: 2 in, 1 out]
      n210 = Format Into String(format string="#%s#" ("初始字符串"), w372) -> (resulting string=w389:string)  [unwired: 2 in, 1 out]
      n211 = Concatenate Strings("where 参数 ='" ("condition"), w371, "' and 时间 between ", w393, "and" ("字符串"), w389) -> (w381:string)
      n212 = call "SQL查询.vi"("condition"=w381, "table输入"=w377, "database"="database1.mdb") -> ("error out"=w383:errorcluster, "data"=w380:string[][])  [unwired: 7 in]
      n213 = case shown="默认" w377 {
        tunnel: w377 -> [_ w413]
        tunnel: w381 -> [_ w412]
        tunnel: w380 -> [_ w411]
        frame Default {
        }
        frame "CODCr", "总氮", "总磷" {
          n214 = global write "全局 实时数据参数.vi" "data"(w411) -> ()
          n215 = global write "全局 实时数据参数.vi" "参数"(w413) -> ()
          n216 = global write "全局 实时数据参数.vi" "连接的字符串"(w412) -> ()
        }
      }
      n217 = case shown="假" FALSE {
        tunnel: [w415 w418] -> w385
        tunnel: w380 -> [w415 w417]
        tunnel: w383 -> [w414 w416]
        tunnel: [w414 w416] -> w382
        frame False {
        }
        frame True {
          # "数字字符串精度转换保留"
          n218 = Index Array(array=w417, index (col)=3 ("禁用的索引 (列)")) -> (element=w424:string[])  [unwired: 1 in]
          n219 = for {
            tunnel: w424 -> [w427] mode=indexing
            tunnel: [w426] -> w420 mode=indexing
            n220 = Fract/Exp String To Number(string=w427) -> (number=w428:dbl)  [unwired: 3 in, 1 out]
            n221 = Number To Fractional String(number=w428, precision (6)=i16 2 ("精度(6)")) -> (F-format string=w426:string)  [unwired: 2 in]
          }
          n222 = Delete From Array(array=w417, length=1 ("长度"), index (col)=3 ("禁用的索引 (列)")) -> (array with subset deleted=w421:string[][])  [unwired: 1 in, 1 out]
          n223 = Insert Into Array(array=w421, index (col)=3 ("禁用的索引 (列)"), new element=w420) -> (w418:string[][])  [unwired: 1 in]
        }
      }
    }
    frame "提取加标回收" {
      w432 = "加标回收率" ("字符串")
      # "上传本地时间点的实时数据"
      n224 = global read "全局 数据发送重叠.vi" "掉线指示灯"() -> (w433:bool)
      n225 = case shown="假" w433 {
        tunnel: [w449 w453] -> w434
        frame False {
          n226 = global read "全局 数据发送重叠.vi" "数据发送重叠"() -> (w450:bool)
          n227 = case shown="假" w450 {
            tunnel: [w451 w452] -> w449
            frame False {
              n228 = global read "起始时间.vi" "起始时间"() -> (w451:string)
            }
            frame True {
              n229 = global read "全局 数据发送重叠.vi" "数据发送重叠开始时间戳"() -> (w452:string)
            }
          }
        }
        frame True {
          n230 = global read "全局 数据发送重叠.vi" "TCP掉线时间节点"() -> (w453:string)
        }
      }
      n231 = global read "起始时间.vi" "结束时间"() -> (w431:string)
      n232 = Format Into String(format string="#%s#" ("初始字符串"), w434) -> (resulting string=w448:string)  [unwired: 2 in, 1 out]
      n233 = Format Into String(format string="#%s#" ("初始字符串"), w431) -> (resulting string=w444:string)  [unwired: 2 in, 1 out]
      n234 = Concatenate Strings("where 参数 ='" ("condition"), w430, "' and 时间 between ", w448, "and" ("字符串"), w444) -> (w436:string)
      n235 = call "SQL查询.vi"("condition"=w436, "table输入"=w432, "database"="database1.mdb") -> ("error out"=w438:errorcluster, "data"=w435:string[][])  [unwired: 7 in]
      n236 = case shown="\"CODCr\", \"总氮\", \"总磷\"" w432 {
        tunnel: w432 -> [_ w456]
        tunnel: w436 -> [_ w455]
        tunnel: w435 -> [_ w454]
        frame Default {
        }
        frame "CODCr", "总氮", "总磷" {
          n237 = global write "全局 实时数据参数.vi" "data"(w454) -> ()
          n238 = global write "全局 实时数据参数.vi" "参数"(w456) -> ()
          n239 = global write "全局 实时数据参数.vi" "连接的字符串"(w455) -> ()
        }
      }
      n240 = case shown="假" FALSE {
        tunnel: [w458 w461] -> w440
        tunnel: w435 -> [w458 w460]
        tunnel: w438 -> [w457 w459]
        tunnel: [w457 w459] -> w437
        frame False {
        }
        frame True {
          # "数字字符串精度转换保留"
          n241 = Index Array(array=w460, index (col)=3 ("禁用的索引 (列)")) -> (element=w467:string[])  [unwired: 1 in]
          n242 = for {
            tunnel: w467 -> [w470] mode=indexing
            tunnel: [w469] -> w463 mode=indexing
            n243 = Fract/Exp String To Number(string=w470) -> (number=w471:dbl)  [unwired: 3 in, 1 out]
            n244 = Number To Fractional String(number=w471, precision (6)=i16 2 ("精度(6)")) -> (F-format string=w469:string)  [unwired: 2 in]
          }
          n245 = Delete From Array(array=w460, length=1 ("长度"), index (col)=3 ("禁用的索引 (列)")) -> (array with subset deleted=w464:string[][])  [unwired: 1 in, 1 out]
          n246 = Insert Into Array(array=w464, index (col)=3 ("禁用的索引 (列)"), new element=w463) -> (w461:string[][])  [unwired: 1 in]
        }
      }
    }
    frame "提取平行样" {
      w475 = "平行样测试" ("字符串")
      # "上传本地时间点的实时数据"
      n247 = global read "全局 数据发送重叠.vi" "掉线指示灯"() -> (w476:bool)
      n248 = case shown="假" w476 {
        tunnel: [w492 w496] -> w477
        frame False {
          n249 = global read "全局 数据发送重叠.vi" "数据发送重叠"() -> (w493:bool)
          n250 = case shown="假" w493 {
            tunnel: [w494 w495] -> w492
            frame False {
              n251 = global read "起始时间.vi" "起始时间"() -> (w494:string)
            }
            frame True {
              n252 = global read "全局 数据发送重叠.vi" "数据发送重叠开始时间戳"() -> (w495:string)
            }
          }
        }
        frame True {
          n253 = global read "全局 数据发送重叠.vi" "TCP掉线时间节点"() -> (w496:string)
        }
      }
      n254 = global read "起始时间.vi" "结束时间"() -> (w474:string)
      n255 = Format Into String(format string="#%s#" ("初始字符串"), w477) -> (resulting string=w491:string)  [unwired: 2 in, 1 out]
      n256 = Format Into String(format string="#%s#" ("初始字符串"), w474) -> (resulting string=w487:string)  [unwired: 2 in, 1 out]
      n257 = Concatenate Strings("where 参数 ='" ("condition"), w473, "' and 时间 between ", w491, "and" ("字符串"), w487) -> (w479:string)
      n258 = call "SQL查询.vi"("condition"=w479, "table输入"=w475, "database"="database1.mdb") -> ("error out"=w481:errorcluster, "data"=w478:string[][])  [unwired: 7 in]
      n259 = case shown="\"CODCr\", \"总氮\", \"总磷\"" w475 {
        tunnel: w475 -> [_ w499]
        tunnel: w479 -> [_ w498]
        tunnel: w478 -> [_ w497]
        frame Default {
        }
        frame "CODCr", "总氮", "总磷" {
          n260 = global write "全局 实时数据参数.vi" "data"(w497) -> ()
          n261 = global write "全局 实时数据参数.vi" "参数"(w499) -> ()
          n262 = global write "全局 实时数据参数.vi" "连接的字符串"(w498) -> ()
        }
      }
      n263 = case shown="假" FALSE {
        tunnel: [w501 w504] -> w483
        tunnel: w478 -> [w501 w503]
        tunnel: w481 -> [w500 w502]
        tunnel: [w500 w502] -> w480
        frame False {
        }
        frame True {
          # "数字字符串精度转换保留"
          n264 = Index Array(array=w503, index (col)=3 ("禁用的索引 (列)")) -> (element=w510:string[])  [unwired: 1 in]
          n265 = for {
            tunnel: w510 -> [w513] mode=indexing
            tunnel: [w512] -> w506 mode=indexing
            n266 = Fract/Exp String To Number(string=w513) -> (number=w514:dbl)  [unwired: 3 in, 1 out]
            n267 = Number To Fractional String(number=w514, precision (6)=i16 2 ("精度(6)")) -> (F-format string=w512:string)  [unwired: 2 in]
          }
          n268 = Delete From Array(array=w503, length=1 ("长度"), index (col)=3 ("禁用的索引 (列)")) -> (array with subset deleted=w507:string[][])  [unwired: 1 in, 1 out]
          n269 = Insert Into Array(array=w507, index (col)=3 ("禁用的索引 (列)"), new element=w506) -> (w504:string[][])  [unwired: 1 in]
        }
      }
    }
    frame "提取集成干预" {
      w518 = "集成干预测试" ("字符串")
      # "上传本地时间点的实时数据"
      n270 = global read "全局 数据发送重叠.vi" "掉线指示灯"() -> (w519:bool)
      n271 = case shown="假" w519 {
        tunnel: [w535 w539] -> w520
        frame False {
          n272 = global read "全局 数据发送重叠.vi" "数据发送重叠"() -> (w536:bool)
          n273 = case shown="假" w536 {
            tunnel: [w537 w538] -> w535
            frame False {
              n274 = global read "起始时间.vi" "起始时间"() -> (w537:string)
            }
            frame True {
              n275 = global read "全局 数据发送重叠.vi" "数据发送重叠开始时间戳"() -> (w538:string)
            }
          }
        }
        frame True {
          n276 = global read "全局 数据发送重叠.vi" "TCP掉线时间节点"() -> (w539:string)
        }
      }
      n277 = global read "起始时间.vi" "结束时间"() -> (w517:string)
      n278 = Format Into String(format string="#%s#" ("初始字符串"), w520) -> (resulting string=w534:string)  [unwired: 2 in, 1 out]
      n279 = Format Into String(format string="#%s#" ("初始字符串"), w517) -> (resulting string=w530:string)  [unwired: 2 in, 1 out]
      n280 = Concatenate Strings("where 参数 ='" ("condition"), w516, "' and 时间 between ", w534, "and" ("字符串"), w530) -> (w522:string)
      n281 = call "SQL查询.vi"("condition"=w522, "table输入"=w518, "database"="database1.mdb") -> ("error out"=w524:errorcluster, "data"=w521:string[][])  [unwired: 7 in]
      n282 = case shown="\"CODCr\", \"总氮\", \"总磷\"" w518 {
        tunnel: w518 -> [_ w542]
        tunnel: w522 -> [_ w541]
        tunnel: w521 -> [_ w540]
        frame Default {
        }
        frame "CODCr", "总氮", "总磷" {
          n283 = global write "全局 实时数据参数.vi" "data"(w540) -> ()
          n284 = global write "全局 实时数据参数.vi" "参数"(w542) -> ()
          n285 = global write "全局 实时数据参数.vi" "连接的字符串"(w541) -> ()
        }
      }
      n286 = case shown="假" FALSE {
        tunnel: [w544 w547] -> w526
        tunnel: w521 -> [w544 w546]
        tunnel: w524 -> [w543 w545]
        tunnel: [w543 w545] -> w523
        frame False {
        }
        frame True {
          # "数字字符串精度转换保留"
          n287 = Index Array(array=w546, index (col)=3 ("禁用的索引 (列)")) -> (element=w553:string[])  [unwired: 1 in]
          n288 = for {
            tunnel: w553 -> [w556] mode=indexing
            tunnel: [w555] -> w549 mode=indexing
            n289 = Fract/Exp String To Number(string=w556) -> (number=w557:dbl)  [unwired: 3 in, 1 out]
            n290 = Number To Fractional String(number=w557, precision (6)=i16 2 ("精度(6)")) -> (F-format string=w555:string)  [unwired: 2 in]
          }
          n291 = Delete From Array(array=w546, length=1 ("长度"), index (col)=3 ("禁用的索引 (列)")) -> (array with subset deleted=w550:string[][])  [unwired: 1 in, 1 out]
          n292 = Insert Into Array(array=w550, index (col)=3 ("禁用的索引 (列)"), new element=w549) -> (w547:string[][])  [unwired: 1 in]
        }
      }
    }
    frame "提取实时数据" {
      # "上传给定时间段之间的实时数据"
      n293 = global read "起始时间.vi" "起始时间"() -> (w569:string)
      n294 = global read "起始时间.vi" "结束时间"() -> (w568:string)
      n295 = global read "全局 实时数据参数.vi" "实时数据参数"() -> (w561:string)
      n296 = Format Into String(format string="#%s#" ("初始字符串"), w569) -> (resulting string=w576:string)  [unwired: 2 in, 1 out]
      n297 = Format Into String(format string="#%s#" ("初始字符串"), w568) -> (resulting string=w570:string)  [unwired: 2 in, 1 out]
      n298 = Concatenate Strings("where 测量模式 ='" ("condition"), w561, "' and 时间 between ", w576, "and" ("字符串"), w570) -> (w574:string)
      n299 = call "SQL查询.vi"("condition"=w574, "table输入"=w559, "database"="database1.mdb") -> ("error out"=w565:errorcluster, "data"=w567:string[][])  [unwired: 7 in]
      n300 = case shown="假" FALSE {
        tunnel: w567 -> [w578 w586]
        tunnel: [w578 w580] -> w566
        tunnel: w565 -> [w577 w579]
        tunnel: [w577 w579] -> w564
        frame False {
        }
        frame True {
          # "数字字符串精度转换保留"
          n301 = Index Array(array=w586, index (col)=3 ("禁用的索引 (列)")) -> (element=w587:string[])  [unwired: 1 in]
          n302 = for {
            tunnel: w587 -> [w590] mode=indexing
            tunnel: [w589] -> w582 mode=indexing
            n303 = Fract/Exp String To Number(string=w590) -> (number=w591:dbl)  [unwired: 3 in, 1 out]
            n304 = Number To Fractional String(number=w591, precision (6)=i16 2 ("精度(6)")) -> (F-format string=w589:string)  [unwired: 2 in]
          }
          n305 = Delete From Array(array=w586, length=1 ("长度"), index (col)=3 ("禁用的索引 (列)")) -> (array with subset deleted=w583:string[][])  [unwired: 1 in, 1 out]
          n306 = Insert Into Array(array=w583, index (col)=3 ("禁用的索引 (列)"), new element=w582) -> (w580:string[][])  [unwired: 1 in]
        }
      }
    }
  }
  "待发送数据" <- w3
  n307 = call <vilib>:"Clear Errors.vi"("error in (no error)"=w7) -> ("error out"=→"error out":errorcluster)  [unwired: 5 in, 1 out]
  n308 = Index Array(array=w3, index (row)=0 ("索引 (行)")) -> (element=→"待发送第一条数据":string[])  [unwired: 1 in]
